vi "lok_graf.vi"() -> ()   [LabVIEW 2020]
uses:
  <vilib>/numeric/Random Number (Range) DBL.vi
panel:
  in  "stop":bool
  out "Waveform Graph":dbl[][](graph)
  in  "Phase":dbl
  in  "Frekvence 2":dbl
  in  "Pocet vzorku":dbl
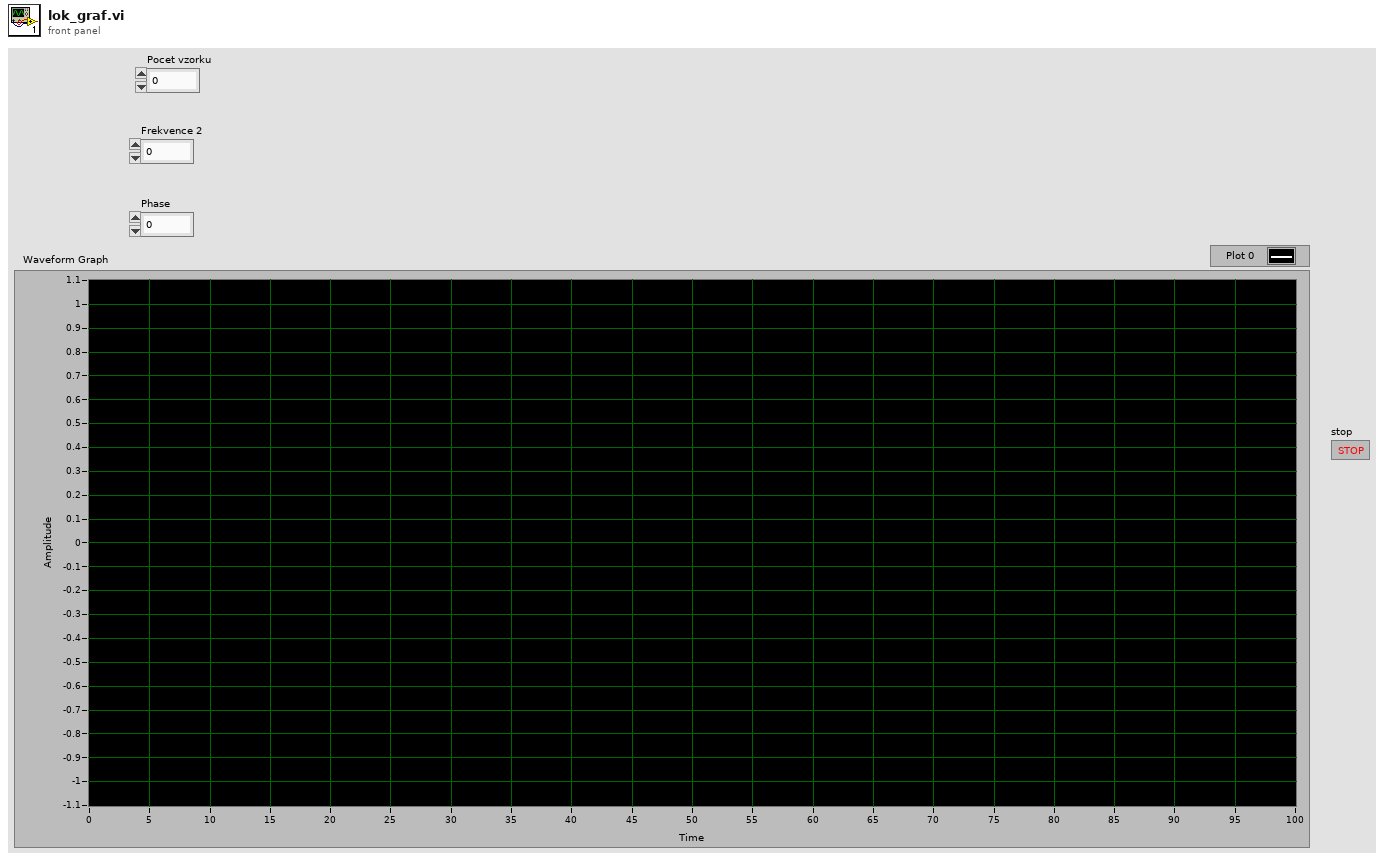
[diagram p1: front panel]
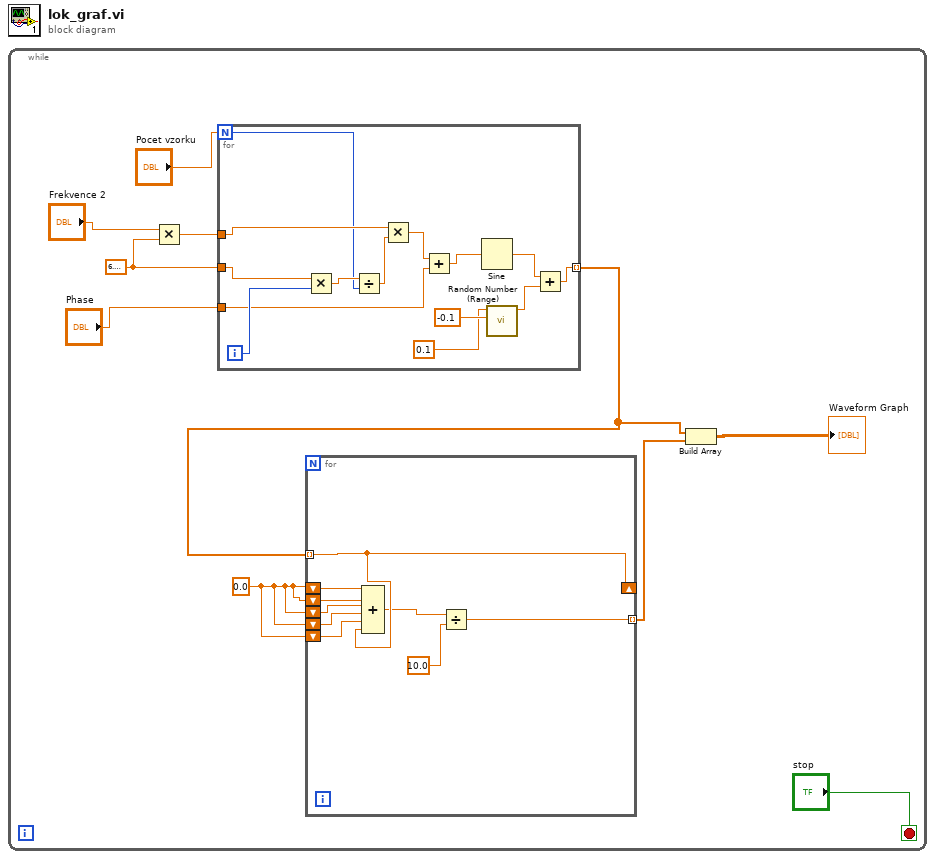
[diagram p0: block diagram]
diagram:
  n1 = while {
    stop <- "stop" stop-if-true
    w5 = 0.0
    w6 = 6.283185307179586
    n2 = Multiply(x="Frekvence 2", y=w6) -> (x*y=w8:dbl)
    n3 = for {
      N: "Pocet vzorku" -> [w27]
      tunnel: w8 -> [w33]
      tunnel: "Phase" -> [w30]
      tunnel: w6 -> [w32]
      tunnel: [w23] -> w4 mode=indexing
      i -> [w31]
      n4 = Multiply(x=w32, y=w31) -> (x*y=w28:dbl)
      n5 = Divide(x=w28, y=w27) -> (x/y=w26:dbl)
      n6 = Multiply(x=w33, y=w26) -> (x*y=w29:dbl)
      n7 = Add(x=w29, y=w30) -> (x+y=w25:dbl)
      n8 = Sine(x=w25) -> (sin(x)=w24:dbl)
      n9 = call-poly <vilib>:"Random Number (Range).vi"("lower bound (0)"=-0.1, "upper bound (100)"=0.1) -> ("number"=w20:dbl)  [unwired: 9 in]
      n10 = Add(x=w24, y=w20) -> (x+y=w23:dbl)
    }
    n11 = for {
      tunnel: w4 -> [w14] mode=indexing
      shift-right: [w14] -> _
      shift-left: w5 -> [w19]
      shift-left: w5 -> [w18]
      shift-left: w5 -> [w17]
      shift-left: w5 -> [w16]
      shift-left: w5 -> [w15]
      tunnel: [w11] -> w3 mode=indexing
      n12 = Compound Arithmetic op=ADD(w19, w18, w17, w16, w15, w14) -> (w13:dbl)
      n13 = Divide(x=w13, y=10.0) -> (x/y=w11:dbl)
    }
    n14 = Build Array(w4, w3) -> (→"Waveform Graph":dbl[][])
  }
